vi "DAQmx.Start AO.vi"(8 "error in (no error)":errorcluster, 11 "DAQmx in":refnum<class "DAQmx.lvclass">) -> (0 "error out":errorcluster, 3 "DAQmx out":refnum<class "DAQmx.lvclass">)   [LabVIEW 2019, in "DAQmx.lvclass"]
uses:
  DAQmx.lvclass
  DAQmx.lvclass/DAQmx.ctl
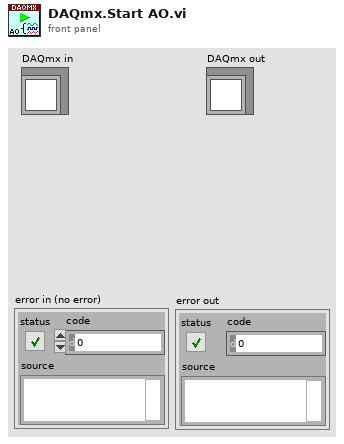
[diagram p1: front panel]
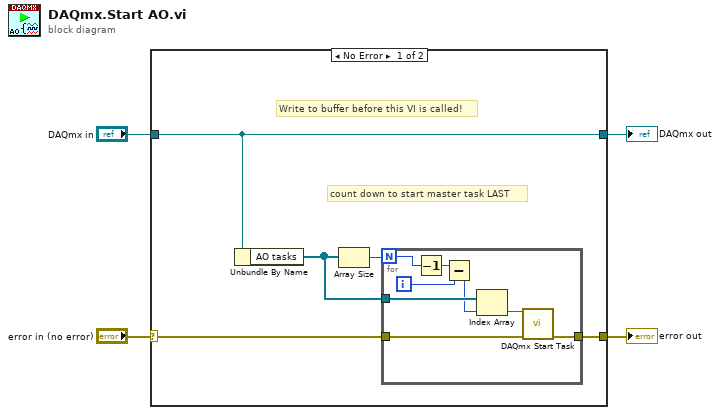
[diagram p0: block diagram]
diagram:
  n1 = case shown="No Error" "error in (no error)" {
    selector: "error in (no error)" -> [w6 w19]
    tunnel: [w9 w19] -> w4
    tunnel: "DAQmx in" -> [w5 w18]
    tunnel: [w5 w18] -> w1
    frame No Error {
      # "Write to buffer before this VI is called!"
      # "count down to start master task LAST"
      n2 = Unbundle By Name(w5) -> ("AO tasks"=w7:refnum<k21>[])
      n3 = Array Size(array=w7) -> (size(s)=w8:i32)
      n4 = for {
        N: w8 -> [w15]
        tunnel: w7 -> [w16]
        tunnel: [w17] -> w9
        tunnel: w6 -> [w11]
        i -> [w12]
        n5 = Decrement(x=w15) -> (x-1=w14:i32)
        n6 = Subtract(x=w14, y=w12) -> (x-y=w13:i32)
        n7 = Index Array(array=w16, index=w13) -> (element=w10:refnum<k21>)
        n8 = call <vilib>:"DAQmx Start Task.vi"("task/channels in"=w10, "error in"=w11) -> ("error out"=w17:errorcluster)  [unwired: 12 in, 1 out]
      }
    }
    frame Error {
    }
  }
  "DAQmx out" <- w1
  "error out" <- w4
